vi "MainView.vi"   [LabVIEW 2016, in "M1M3SupportViews.lvlib"]
uses:
  M1M3SupportViews.lvlib
  UserEvents/UserEvents.lvclass
  Communicator/M1M3SAL/M1M3SAL.lvclass
  Communicator/M1M3SAL/M1M3SAL.lvclass/M1M3SAL.ctl
  UserEvents/UserEvents.lvclass/UserEvents.ctl
  ApplicationStatusView.vi
  ApplicationControlView.vi
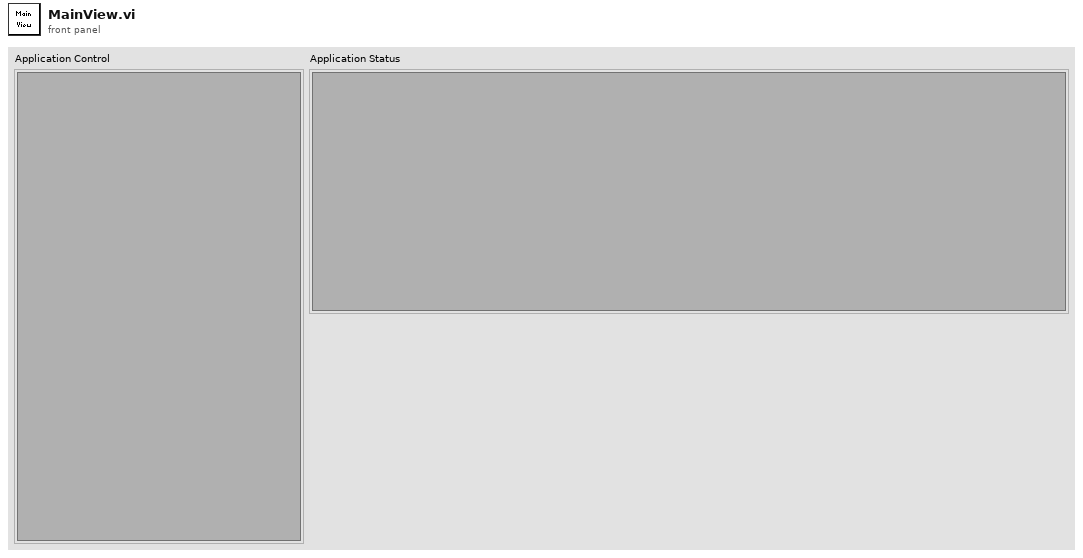
[diagram p1: front panel]
types:
  T1 = enum32{"invalid app kind", "Development System", "Run Time System", "Student Edition", "Embedded LabVIEW", "Evaluation", "Custom"}
  T2 = cluster{"IPAddress":string, "Port":u16, "StartupScript":string}
  T3 = cluster{"Application Control":refnum<vi>, refnum<vi>}
  T4 = cluster{"Application Status":refnum<vi>, refnum<vi>}
  T5 = cluster{"Application Status":refnum<vi>, refnum<vi>}[]
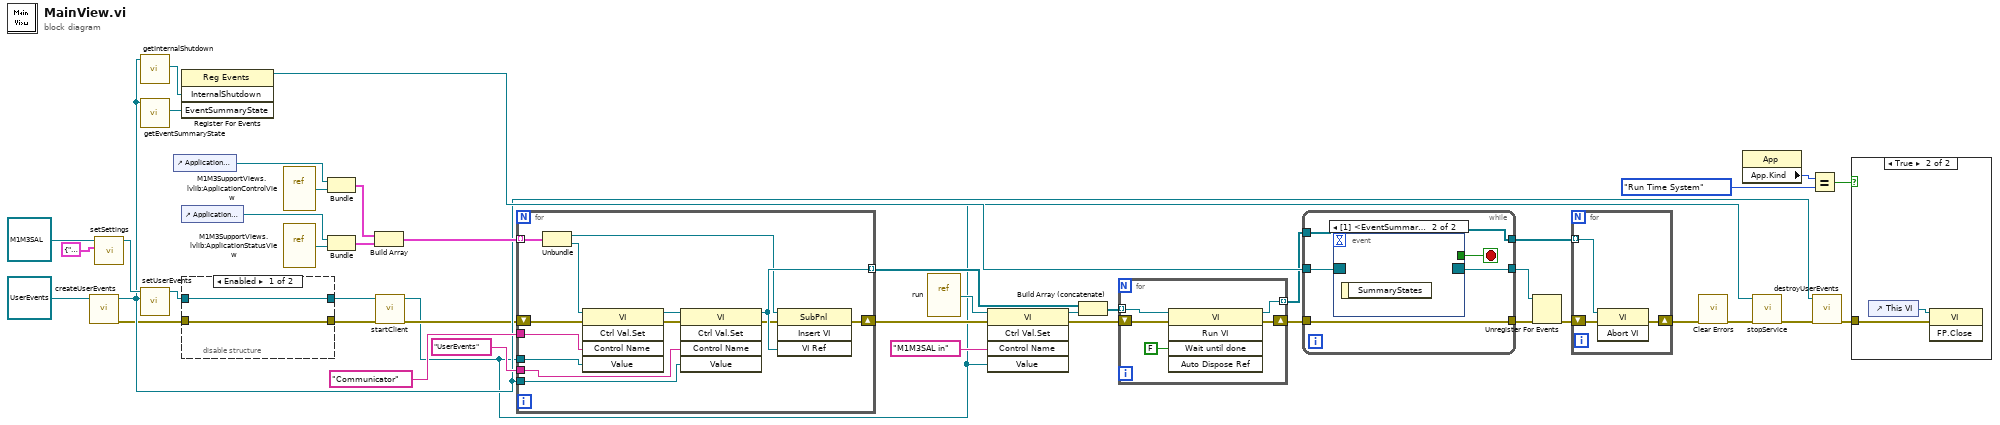
[diagram p0: block diagram]
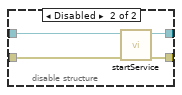
[diagram p2: hidden frame]
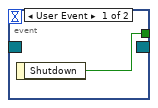
[diagram p4: hidden frame]
diagram:
  n1 = call "createUserEvents.vi"("UserEvents in"=refnum<class "UserEvents.lvclass"> refnum ("UserEvents.lvclass")) -> ("error out"=w8:errorcluster, "UserEvents out"=w20:refnum<class "UserEvents.lvclass">)  [unwired: 9 in]
  n2 = call "setSettings.vi"("Settings"=T2 {"IPAddress"="140.252.24.118", "Port"=5020, "StartupScript"="source /usr/ts_sal/setup.env && /usr/ts_sal/test/m1m3/cpp/src/SALPipe %d -1"}, "M1M3SAL in"=refnum<class "M1M3SAL.lvclass"> refnum ("M1M3Communicator.lvlib:M1M3SAL.lvclass")) -> ("M1M3SAL out"=w38:refnum<class "M1M3SAL.lvclass">)  [unwired: 9 in]
  n3 = call "getInternalShutdown.vi"("UserEvents in"=w20) -> ("InternalShutdown"=w36:refnum<user-event>)  [unwired: 9 in, 1 out]
  n4 = call "getEventSummaryState.vi"("UserEvents in"=w20) -> ("EventSummaryState"=w35:refnum<user-event>)  [unwired: 9 in, 1 out]
  n5 = call "setUserEvents.vi"("UserEvents"=w20, "M1M3SAL in"=w38) -> ("M1M3SAL out"=w9:refnum<class "M1M3SAL.lvclass">)  [unwired: 9 in]
  n6 = control-ref of="Application Control"() -> (w12:refnum<vi>)
  n7 = register-events(w36, w35) -> (reference out=w34:refnum<event-registration>)  [unwired: 2 in, 1 out]
  n8 = control-ref of="Application Status"() -> (w11:refnum<vi>)
  n9 = disable-structure shown="Enabled" {
    disable-tunnel: w9 -> [w45 w49]
    disable-tunnel: [w45 w47] -> w7
    disable-tunnel: w8 -> [w44 w48]
    disable-tunnel: [w44 w46] -> w6
    frame Enabled {
    }
    frame Disabled {
      n10 = call-dynamic "startService.vi"("error in (no error)"=w48, "M1M3SAL in"=w49) -> ("error out"=w46:errorcluster, "M1M3SAL out"=w47:refnum<class "M1M3SAL.lvclass">)  [unwired: 8 in]
    }
  }
  n11 = vi-ref "M1M3SupportViews.lvlib:ApplicationControlView.vi"() -> (w13:refnum<vi>)
  n12 = vi-ref "M1M3SupportViews.lvlib:ApplicationStatusView.vi"() -> (w27:refnum<vi>)
  n13 = Bundle("Application Control"=w12, w13) -> (w26:T3)  [unwired: 1 in]
  n14 = Bundle("Application Status"=w11, w27) -> (w25:T4)  [unwired: 1 in]
  n15 = Build Array(w26, w25) -> (w43:T5)
  n16 = call-dynamic "startClient.vi"("error in (no error)"=w6, "M1M3SAL in"=w7) -> ("error out"=w5:errorcluster, "M1M3SAL out"=w3:refnum<class "M1M3SAL.lvclass">)  [unwired: 8 in]
  n17 = for {
    tunnel: w43 -> [w52] mode=indexing
    tunnel: "Communicator" -> [w60]
    tunnel: "UserEvents" -> [w59]
    tunnel: w20 -> [w58]
    tunnel: w3 -> [w57]
    tunnel: [w56] -> w19 mode=indexing
    shift-right: [w53] -> w10
    shift-left: w5 -> [w55]
    n18 = Unbundle(w52) -> ("Application Status"=w50:refnum<vi>, w51:refnum<vi>)
    n19 = invoke class="VI" method="Ctrl Val.Set"(reference=w51, error in=w55, "Control Name"=w60, "Value"=w57) -> (reference out=w62:refnum<vi>, error out=w61:errorcluster)  [unwired: 1 in, 3 out]
    n20 = invoke class="VI" method="Ctrl Val.Set"(reference=w62, error in=w61, "Control Name"=w59, "Value"=w58) -> (reference out=w56:refnum<vi>, error out=w54:errorcluster)  [unwired: 1 in, 3 out]
    n21 = invoke class="SubPnl" method="Insert VI"(reference=w50, error in=w54, "VI Ref"=w56) -> (error out=w53:errorcluster)  [unwired: 1 in, 3 out]
  }
  n22 = vi-ref "run.vi"() -> (w17:refnum<vi>)
  n23 = invoke class="VI" method="Ctrl Val.Set"(reference=w17, error in=w10, "Control Name"="M1M3SAL in", "Value"=w3) -> (reference out=w15:refnum<vi>, error out=w14:errorcluster)  [unwired: 1 in, 3 out]
  n24 = Build Array (concatenate)(w19, w15) -> (w18:refnum<vi>[])
  n25 = for {
    tunnel: w18 -> [w67] mode=indexing
    tunnel: [w65] -> w33 mode=indexing
    shift-right: [w63] -> w29
    shift-left: w14 -> [w64]
    n26 = invoke class="VI" method="Run VI"(reference=w67, error in=w64, "Wait until done"=FALSE ("Wait Until Done")) -> (reference out=w65:refnum<vi>, error out=w63:errorcluster)  [unwired: 2 in, 3 out]
  }
  n27 = while {
    tunnel: w34 -> [w72]
    tunnel: w33 -> [w70]
    tunnel: [w70] -> w31
    tunnel: [w69] -> w32
    tunnel: w29 -> [w68]
    tunnel: [w68] -> w28
    stop <- w71 stop-if-true
    n28 = event shown="[1] <EventSummaryState>: User Event" {
      selector: w72 -> [_ _]
      dyn-events: [_ _] -> w69
      timeout: _ -> [_ _]
      tunnel: [w73 _] -> w71
      event User Event {
        n29 = event-data() -> ("Shutdown"=w73:bool)  [unwired: 1 in]
      }
      event User Event {
        n30 = event-data() -> ()  [unwired: 1 in, 1 out]
      }
    }
  }
  n31 = Unregister For Events(event registration refnum=w32, error in=w28) -> (error out=w30:errorcluster)
  n32 = for {
    tunnel: w31 -> [w76] mode=indexing
    shift-right: [w74] -> w2
    shift-left: w30 -> [w75]
    n33 = invoke class="VI" method="Abort VI"(reference=w76, error in=w75) -> (error out=w74:errorcluster)  [unwired: 1 in, 2 out]
  }
  n34 = call <vilib>:"Clear Errors.vi"("error in (no error)"=w2) -> ("error out"=w1:errorcluster)  [unwired: 5 in, 1 out]
  n35 = property class="App"() -> ("App.Kind"=w24:T1)  [unwired: 2 in, 2 out]
  n36 = call-dynamic "stopService.vi"("error in (no error)"=w1, "M1M3SAL in"=w3) -> ("error out"=w4:errorcluster)  [unwired: 8 in, 1 out]
  n37 = Equal?(x=w24, y=T1."Run Time System") -> (x = y?=w22:bool)
  n38 = call "destroyUserEvents.vi"("error in (no error)"=w4, "UserEvents in"=w20) -> ("error out"=w21:errorcluster)  [unwired: 8 in, 1 out]
  n39 = case shown="True" w22 {
    tunnel: w21 -> [_ w77]
    frame False {
    }
    frame True {
      n40 = control-ref of="This VI"() -> (w78:refnum<vi>)
      n41 = invoke class="VI" method="FP.Close"(reference=w78, error in=w77) -> ()  [unwired: 1 in, 3 out]
    }
  }
